vi "InsetAndLocalizeRect.vi"(10 "inset params":T1, 11 "rect":T1) -> (3 "local inscribed":T1)   [LabVIEW 2020, in "Cls_AggHandler.xnode"]
uses:
  <vilib>/Utility/AggHandler/Cls_AggHandler.xnode
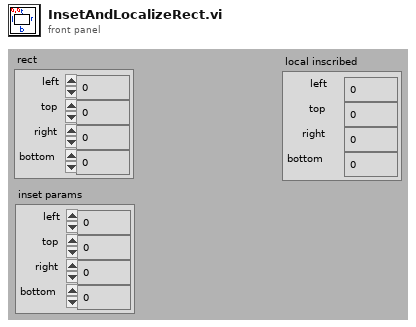
[diagram p1: front panel]
types:
  T1 = cluster{"left":i16, "top":i16, "right":i16, "bottom":i16}
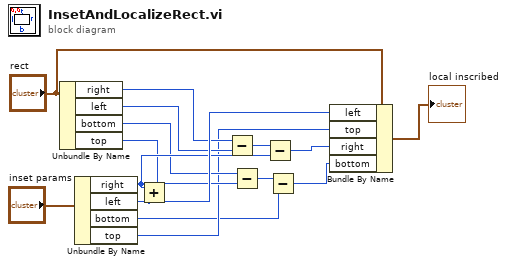
[diagram p0: block diagram]
diagram:
  n1 = Unbundle By Name("rect") -> ("right"=w11:i16, "left"=w10:i16, "bottom"=w6:i16, "top"=w5:i16)
  n2 = Unbundle By Name("inset params") -> ("right"=w8:i16, "left"=w12:i16, "bottom"=w1:i16, "top"=w2:i16)
  n3 = Add(x=w8, y=w12) -> ()  [unwired: 1 out]
  n4 = Subtract(x=w11, y=w10) -> (x-y=w9:i16)
  n5 = Subtract(x=w6, y=w5) -> (x-y=w4:i16)
  n6 = Subtract(x=w9, y=w8) -> (x-y=w7:i16)
  n7 = Subtract(x=w4, y=w1) -> (x-y=w3:i16)
  n8 = Bundle By Name(cluster="rect", "left"=w12, "top"=w2, "right"=w7, "bottom"=w3) -> (→"local inscribed":T1)
